vi "magnet.vi"(1 "resistance":dbl) -> (0 "temperature, K":dbl)   [LabVIEW 2013]
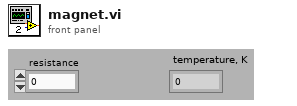
[diagram p1: front panel]
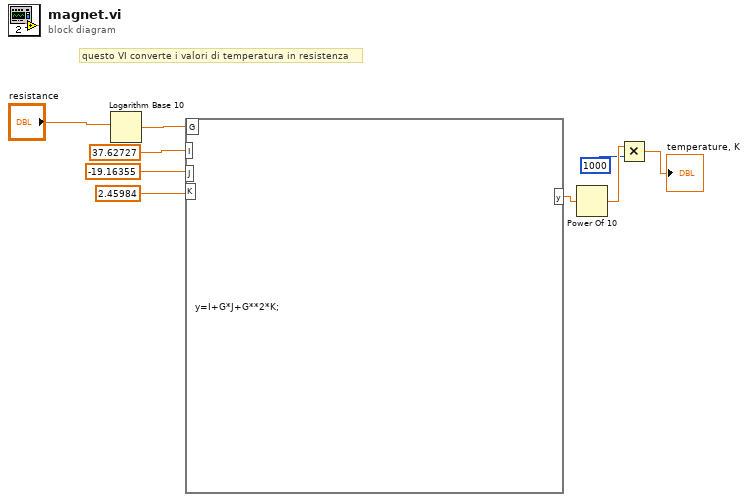
[diagram p0: block diagram]
diagram:
  # "questo VI converte i valori di temperatura in resistenza"
  n1 = Logarithm Base 10(1:"resistance") -> (0:w9:dbl)
  n2 = formula code="y=I+G*J+G**2*K;"("G"=w9, "I"=37.62727 ("input variable"), "J"=-19.16355 ("input variable"), "K"=2.45984 ("input variable")) -> ("y"=w4:dbl)
  n3 = Power Of 10(x=w4) -> (10^x=w3:dbl)
  n4 = Multiply(x=w3, y=1000) -> (x*y=→"temperature, K":dbl)
